vi "Read configuration.vi"(8 "error in (no error)":errorcluster, 11 "Abstract Scope":refnum<class "Scope Instrument.lvclass">) -> (0 "error out":errorcluster, 2 "configuration":refnum<class "CEF_serializable configuration.lvclass">, 3 "Abstract Scope out":refnum<class "Scope Instrument.lvclass">)   [LabVIEW 2025, in "Scope.lvlib" / "Scope Instrument.lvclass"]
uses:
  Scope Instrument.lvclass
  Users/Public/Documents/Sandia National Labs/TSS Plugin/CEF.lvlibp/serializable configuration/CEF_serializable configuration.lvclass
  Scope Instrument.lvclass/Scope Instrument.ctl
  Scope configuration/Scope configuration.lvclass
  C:/Users/Public/Documents/Sandia National Labs/TSS Plugin/CEF.lvlibp/serializable configuration/CEF_serializable configuration.lvclass
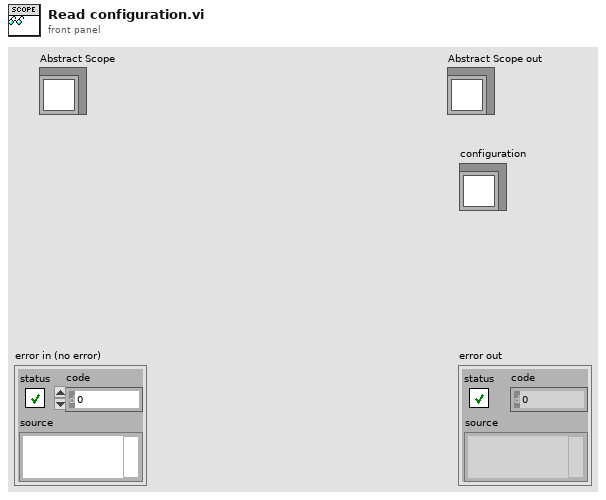
[diagram p1: front panel]
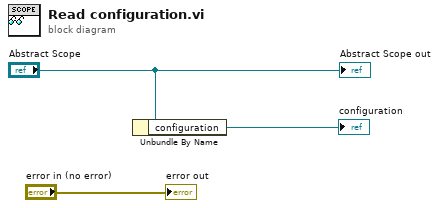
[diagram p0: block diagram]
diagram:
  n1 = Unbundle By Name("Abstract Scope") -> ("configuration"=→"configuration":refnum<class "Scope configuration.lvclass">)
  "error out" <- "error in (no error)"
  "Abstract Scope out" <- "Abstract Scope"
